vi "Autonomous Independent.vi"() -> ()   [LabVIEW 2016]
doc: "This VI is called when autonomous begins, and will automatically be terminated when autonomous ends. You can carry out timed or sensor driven robot movement independently without needing to return to the caller."
uses:
  <vilib>/Rock Robotics/WPI/Utilities/WPI_GetSetVariantRefNum.vi
  <vilib>/Rock Robotics/Network Tables/NT Read String.vi
  SubSystems/References/Refnums.vi
  <vilib>/Rock Robotics/WPI/RobotDrive/WPI_RobotDriveArcadeDrive_Standard(NoSaturation).vi
  <vilib>/Rock Robotics/Network Tables/NT Write Numeric Array.vi
panel:
  out "Motor Output 2":dbl
  out "Motor Output":dbl
  out "inside timer value 2":u32
  out "Current Movement, for debugging":T1 {"Y Joystick Value" scale=1.0..-1.0; "X Joystick Value" scale=-1.0..1.0}
  in  "Array of robot movements":T2(array[cluster])=[{"X Joystick Value"=0.39393939393939403, "Y Joystick Value"=0.0, "Delay (sec)"=1.0, "Movement Name"="turn"}, {"X Joystick Value"=-0.3737373737373737, "Y Joystick Value"=0.0, "Delay (sec)"=1.0, "Movement Name"="turn back"}] {"Y Joystick Value" scale=1.0..-1.0; "X Joystick Value" scale=-1.0..1.0}
  # "Be sure to right-click and choose Data Operations>>Make Current Value default if you want to save the array values with the VI"
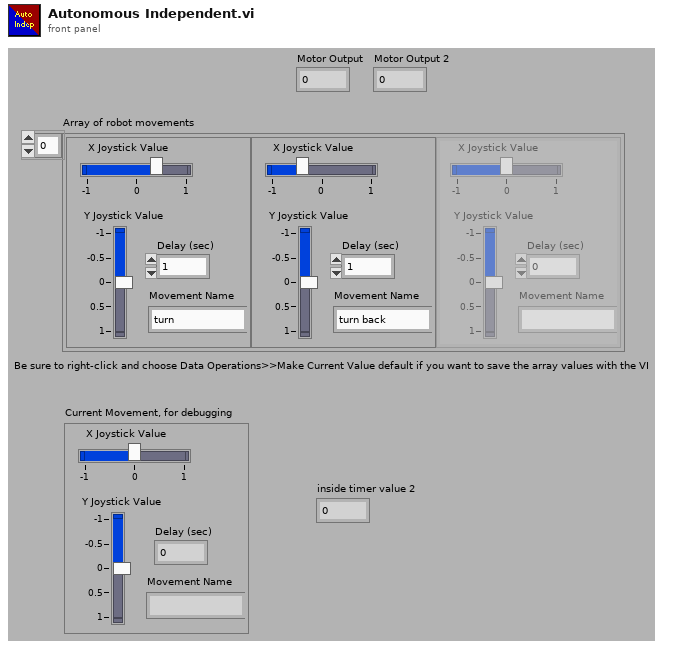
[diagram p1: front panel]
types:
  T1 = cluster{"X Joystick Value":dbl, "Y Joystick Value":dbl, "Delay (sec)":dbl, "Movement Name":string}
  T2 = cluster{"X Joystick Value":dbl, "Y Joystick Value":dbl, "Delay (sec)":dbl, "Movement Name":string}[]
  T3 = typedef "WPI_JoystickDevRef.ctl" = cluster{"Device":T4}
  T4 = typedef "WPI_JoystickDeviceEnum.ctl" = enum16{"USB 0", "USB 1", "USB 2", "USB 3", "USB 4", "USB 5"}
  T5 = typedef "WPI_MotorControlDeviceRef.ctl" = cluster{"DeviceStatus":errorcluster, "Type":T6, "PWM":cluster{"PWM Channel":T7, "DeadBand":T8}, "CAN":cluster{"Device Number":u8, "SetOutput VI Ref":variant, "GetOutput VI Ref":variant, "Enable VI Ref":variant, "Disable VI Ref":variant, "Data":variant}, "Invert":bool}
  T6 = typedef "WPI_MotorControlType.ctl" = enum16{"PWM", "CAN"}
  T7 = typedef "FPGA_DIOPWMChannel.ctl" = enum8{"PWM 0", "PWM 1", "PWM 2", "PWM 3", "PWM 4", "PWM 5", "PWM 6", "PWM 7", "PWM 8", "PWM 9", "PWM MXP 0", "PWM MXP 1", "PWM MXP 2", "PWM MXP 3", "PWM MXP 4", "PWM MXP 5", "PWM MXP 6", "PWM MXP 7", "PWM MXP 8", "PWM MXP 9", "Invalid"}
  T8 = typedef "WPI_PWMDeadband.ctl" = cluster{"Name":string, "maxPositivePwm":i32, "minPositivePwm":i32, "centerPwm":i32, "maxNegativePwm":i32, "minNegativePwm":i32, "angularRange":u16}
  T9 = typedef "WPI_RobotDriveDevRef.ctl" = cluster{"DevStatus":errorcluster, "Motors[]":T5[], "Square Inputs":bool, "Max Output":dbl}
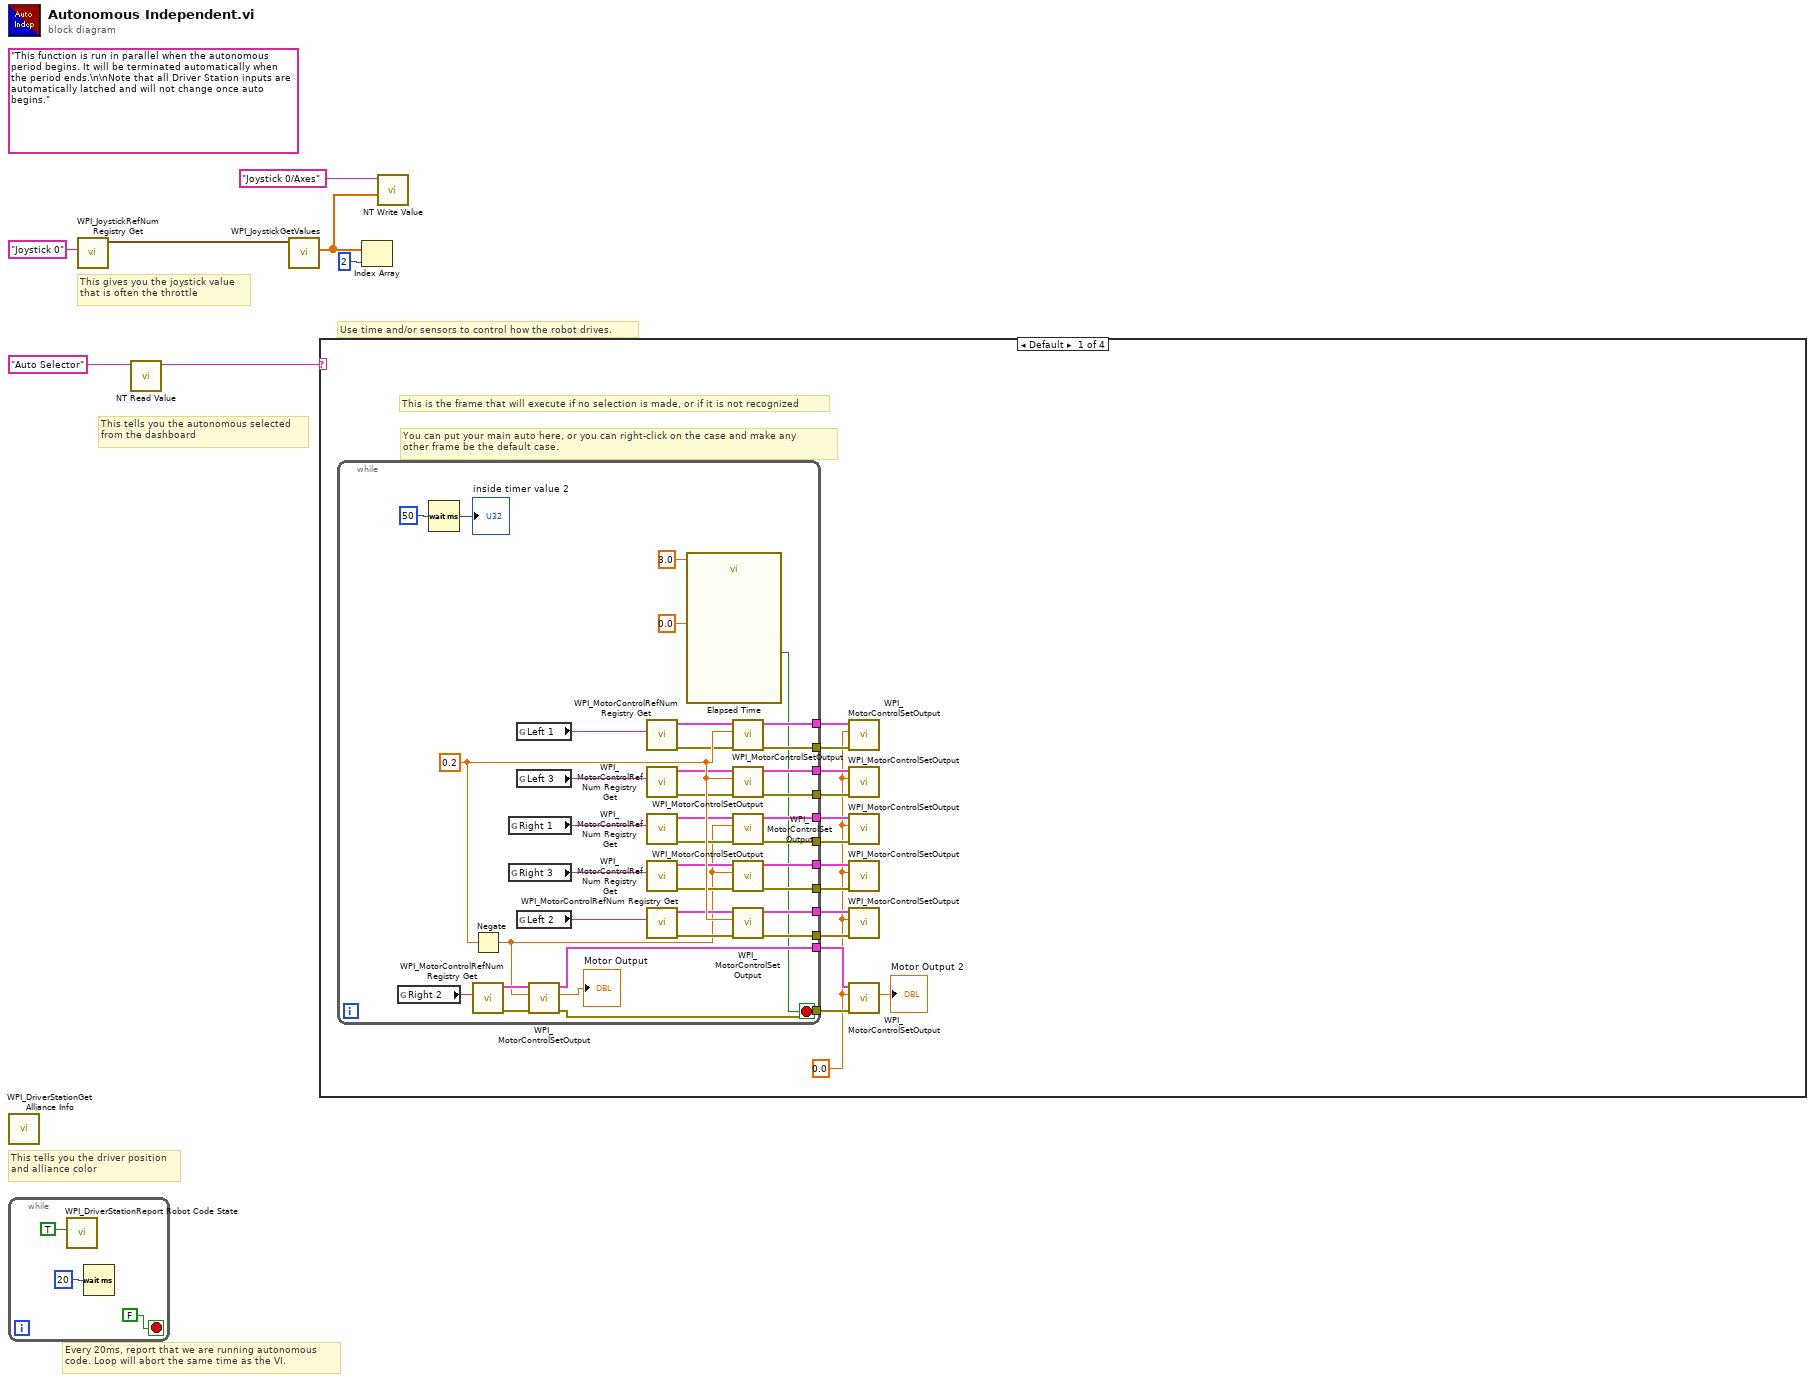
[diagram p0: block diagram]
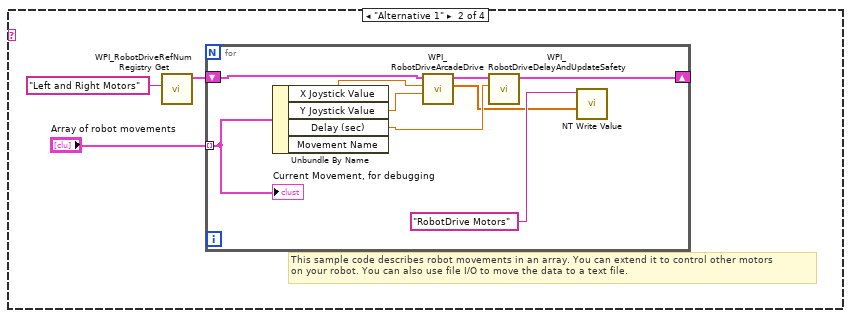
[diagram p2: hidden frame]
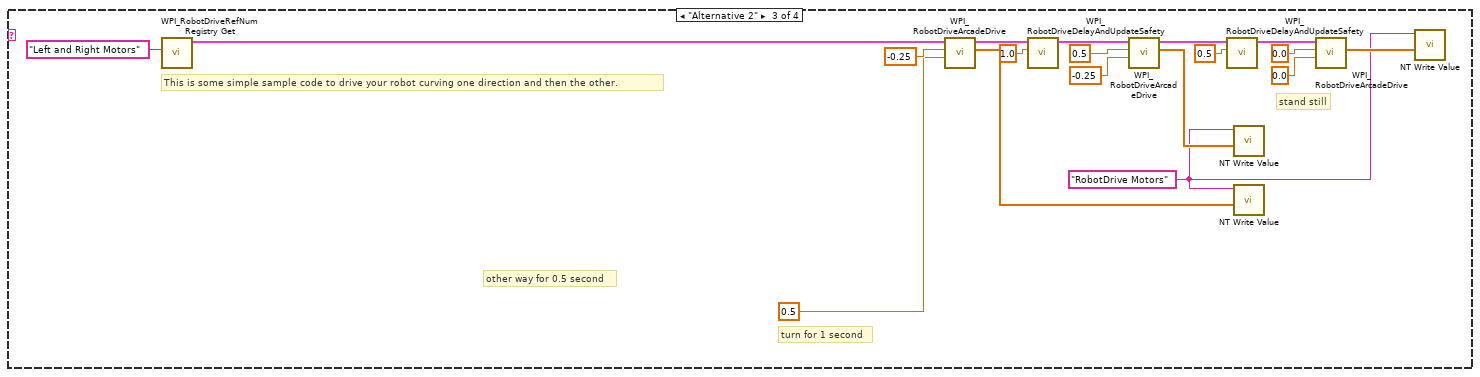
[diagram p3: hidden frame]
diagram:
  (unwired) "This function is run in parallel when the autonomous period begins. It will be terminated automatically when the period ends.\n\nNote that all Driver Station inputs are automatically latched and will not change once auto begins."
  # "This tells you the autonomous selected\nfrom the dashboard"
  # "Every 20ms, report that we are running autonomous\ncode. Loop will abort the same time as the VI."
  # "This gives you the joystick value\nthat is often the throttle"
  # "Use time and/or sensors to control how the robot drives."
  # "This tells you the driver position\nand alliance color"
  n1 = call <vilib>:"WPI_DriverStationGet Alliance Info.vi"() -> ()  [unwired: 12 out]
  n2 = while {
    stop <- FALSE stop-if-true
    n3 = call <vilib>:"WPI_DriverStationReport Robot Code State.vi"("Autonomous"=TRUE) -> ()  [unwired: 10 in, 1 out]
    n4 = Wait (ms)(milliseconds to wait=u32 20) -> ()  [unwired: 1 out]
  }
  n5 = call <vilib>:"WPI_JoystickRefNum Registry Get.vi"("refnum name"="Joystick 0") -> ("JoystickDevRef"=w6:T3)  [unwired: 1 in, 9 out]
  n6 = call-poly <vilib>:"NT Read Value.vi"("Name"="Auto Selector") -> ("String"=w3:string)  [unwired: 9 in, 1 out]
  n7 = call <vilib>:"WPI_JoystickGetValues.vi"("JoystickDevRef"=w6) -> ("Axes"=w2:dbl[])  [unwired: 6 in, 4 out]
  n8 = case shown="Default" w3 {
    frame Default {
      w12 = 0.0 ("Output")
      # "You can put your main auto here, or you can right-click on the case and make any\nother frame be the default case."
      # "This is the frame that will execute if no selection is made, or if it is not recognized"
      n9 = while {
        tunnel: [w40] -> w24
        tunnel: [w39] -> w23
        tunnel: [w38] -> w22
        tunnel: [w37] -> w21
        tunnel: [w36] -> w20
        tunnel: [w35] -> w19
        tunnel: [w34] -> w18
        tunnel: [w33] -> w17
        tunnel: [w32] -> w16
        tunnel: [w31] -> w15
        tunnel: [w30] -> w14
        tunnel: [w29] -> w13
        stop <- w28 stop-if-true
        w61 = 0.2 ("x")
        n10 = global read "Refnums.vi" "Right 2"() -> (w57:string)
        n11 = Wait (ms)(milliseconds to wait=u32 50) -> (millisecond timer value=→"inside timer value 2":u32)
        n12 = Negate(x=w61) -> (-x=w43:dbl)
        n13 = call <vilib>:"WPI_MotorControlRefNum Registry Get.vi"("refnum name"=w57) -> ("error out"=w55:errorcluster, "MotorControlDevRef"=w56:T5)  [unwired: 9 in]
        n14 = global read "Refnums.vi" "Right 1"() -> (w58:string)
        n15 = global read "Refnums.vi" "Right 3"() -> (w52:string)
        n16 = global read "Refnums.vi" "Left 1"() -> (w45:string)
        n17 = global read "Refnums.vi" "Left 3"() -> (w51:string)
        n18 = global read "Refnums.vi" "Left 2"() -> (w46:string)
        n19 = call <vilib>:"WPI_MotorControlSetOutput.vi"("error in (no error)"=w55, "Output"=w43, "MotorControlDevRef"=w56) -> ("error out"=w30:errorcluster, "Motor Output"=→"Motor Output":dbl, "MotorControlDevRef"=w36:T5)  [unwired: 6 in]
        n20 = call <vilib>:"WPI_MotorControlRefNum Registry Get.vi"("refnum name"=w45) -> ("error out"=w44:errorcluster, "MotorControlDevRef"=w42:T5)  [unwired: 9 in]
        n21 = call <vilib>:"WPI_MotorControlRefNum Registry Get.vi"("refnum name"=w51) -> ("error out"=w49:errorcluster, "MotorControlDevRef"=w50:T5)  [unwired: 9 in]
        n22 = call <vilib>:"WPI_MotorControlRefNum Registry Get.vi"("refnum name"=w58) -> ("error out"=w60:errorcluster, "MotorControlDevRef"=w59:T5)  [unwired: 9 in]
        n23 = call <vilib>:"WPI_MotorControlRefNum Registry Get.vi"("refnum name"=w52) -> ("error out"=w54:errorcluster, "MotorControlDevRef"=w53:T5)  [unwired: 9 in]
        n24 = call <vilib>:"WPI_MotorControlRefNum Registry Get.vi"("refnum name"=w46) -> ("error out"=w48:errorcluster, "MotorControlDevRef"=w47:T5)  [unwired: 9 in]
        n25 = call "Elapsed Time"("Time Target (s)"=3.0, "Set Start Time (s)"=0.0) -> ("Time has Elapsed"=w28:bool)  [unwired: 10 in, 7 out]
        n26 = call <vilib>:"WPI_MotorControlSetOutput.vi"("error in (no error)"=w44, "Output"=w61, "MotorControlDevRef"=w42) -> ("error out"=w33:errorcluster, "MotorControlDevRef"=w40:T5)  [unwired: 6 in, 1 out]
        n27 = call <vilib>:"WPI_MotorControlSetOutput.vi"("error in (no error)"=w49, "Output"=w61, "MotorControlDevRef"=w50) -> ("error out"=w34:errorcluster, "MotorControlDevRef"=w38:T5)  [unwired: 6 in, 1 out]
        n28 = call <vilib>:"WPI_MotorControlSetOutput.vi"("error in (no error)"=w60, "Output"=w43, "MotorControlDevRef"=w59) -> ("error out"=w31:errorcluster, "MotorControlDevRef"=w37:T5)  [unwired: 6 in, 1 out]
        n29 = call <vilib>:"WPI_MotorControlSetOutput.vi"("error in (no error)"=w54, "Output"=w43, "MotorControlDevRef"=w53) -> ("error out"=w32:errorcluster, "MotorControlDevRef"=w35:T5)  [unwired: 6 in, 1 out]
        n30 = call <vilib>:"WPI_MotorControlSetOutput.vi"("error in (no error)"=w48, "Output"=w61, "MotorControlDevRef"=w47) -> ("error out"=w29:errorcluster, "MotorControlDevRef"=w39:T5)  [unwired: 6 in, 1 out]
      }
      n31 = call <vilib>:"WPI_MotorControlSetOutput.vi"("error in (no error)"=w17, "Output"=w12, "MotorControlDevRef"=w24) -> ()  [unwired: 6 in, 3 out]
      n32 = call <vilib>:"WPI_MotorControlSetOutput.vi"("error in (no error)"=w18, "Output"=w12, "MotorControlDevRef"=w22) -> ()  [unwired: 6 in, 3 out]
      n33 = call <vilib>:"WPI_MotorControlSetOutput.vi"("error in (no error)"=w15, "Output"=w12, "MotorControlDevRef"=w21) -> ()  [unwired: 6 in, 3 out]
      n34 = call <vilib>:"WPI_MotorControlSetOutput.vi"("error in (no error)"=w16, "Output"=w12, "MotorControlDevRef"=w19) -> ()  [unwired: 6 in, 3 out]
      n35 = call <vilib>:"WPI_MotorControlSetOutput.vi"("error in (no error)"=w13, "Output"=w12, "MotorControlDevRef"=w23) -> ()  [unwired: 6 in, 3 out]
      n36 = call <vilib>:"WPI_MotorControlSetOutput.vi"("error in (no error)"=w14, "Output"=w12, "MotorControlDevRef"=w20) -> ("Motor Output"=→"Motor Output 2":dbl)  [unwired: 6 in, 2 out]
    }
    frame "Alternative 1" {
      # "This sample code describes robot movements in an array. You can extend it to control other motors\non your robot. You can also use file I/O to move the data to a text file."
      n37 = call <vilib>:"WPI_RobotDriveRefNum Registry Get.vi"("refnum name"="Left and Right Motors") -> ("RobotDriveDevRef"=w64:T9)  [unwired: 1 in, 9 out]
      n38 = for {
        shift-right: [w72] -> _
        shift-left: w64 -> [w73]
        tunnel: "Array of robot movements" -> [w68] mode=indexing
        n39 = Unbundle By Name(w68) -> ("X Joystick Value"=w71:dbl, "Y Joystick Value"=w70:dbl, "Delay (sec)"=w69:dbl)  [unwired: 1 out]
        n40 = call-poly <vilib>:"WPI_RobotDriveArcadeDrive.vi"("Y axis value"=w70, "X axis value"=w71, "RobotDriveDevRef"=w73) -> ("Motor Values"=w66:dbl[], "RobotDriveDevRef"=w74:T9)  [unwired: 1 in, 6 out]
        n41 = call <vilib>:"WPI_RobotDriveDelayAndUpdateSafety.vi"("Delay (s)"=w69, "RobotDriveDevRef"=w74) -> ("RobotDriveDevRef 2"=w72:T9)  [unwired: 8 in, 1 out]
        n42 = call-poly <vilib>:"NT Write Value.vi"("Numeric Array"=w66, "Name"="RobotDrive Motors") -> ()  [unwired: 9 in, 1 out]
        "Current Movement, for debugging" <- w68
      }
    }
    frame "Alternative 2" {
      w76 = "RobotDrive Motors" ("Name")
      # "This is some simple sample code to drive your robot curving one direction and then the other."
      # "stand still"
      # "other way for 0.5 second"
      # "turn for 1 second"
      n43 = call <vilib>:"WPI_RobotDriveRefNum Registry Get.vi"("refnum name"="Left and Right Motors") -> ("RobotDriveDevRef"=w92:T9)  [unwired: 1 in, 9 out]
      n44 = call-poly <vilib>:"WPI_RobotDriveArcadeDrive.vi"("Y axis value"=0.5 ("X axis value"), "X axis value"=-0.25, "RobotDriveDevRef"=w92) -> ("Motor Values"=w75:dbl[], "RobotDriveDevRef"=w85:T9)  [unwired: 1 in, 6 out]
      n45 = call <vilib>:"WPI_RobotDriveDelayAndUpdateSafety.vi"("Delay (s)"=1.0, "RobotDriveDevRef"=w85) -> ("RobotDriveDevRef 2"=w86:T9)  [unwired: 8 in, 1 out]
      n46 = call-poly <vilib>:"WPI_RobotDriveArcadeDrive.vi"("Y axis value"=-0.25 ("X axis value"), "X axis value"=0.5, "RobotDriveDevRef"=w86) -> ("Motor Values"=w77:dbl[], "RobotDriveDevRef"=w87:T9)  [unwired: 1 in, 6 out]
      n47 = call <vilib>:"WPI_RobotDriveDelayAndUpdateSafety.vi"("Delay (s)"=0.5, "RobotDriveDevRef"=w87) -> ("RobotDriveDevRef 2"=w88:T9)  [unwired: 8 in, 1 out]
      n48 = call-poly <vilib>:"NT Write Value.vi"("Numeric Array"=w77, "Name"=w76) -> ()  [unwired: 9 in, 1 out]
      n49 = call-poly <vilib>:"NT Write Value.vi"("Numeric Array"=w75, "Name"=w76) -> ()  [unwired: 9 in, 1 out]
      n50 = call-poly <vilib>:"WPI_RobotDriveArcadeDrive.vi"("Y axis value"=0.0 ("X axis value"), "X axis value"=0.0, "RobotDriveDevRef"=w88) -> ("Motor Values"=w78:dbl[])  [unwired: 1 in, 7 out]
      n51 = call-poly <vilib>:"NT Write Value.vi"("Numeric Array"=w78, "Name"=w76) -> ()  [unwired: 9 in, 1 out]
    }
    frame "Your Turn" {
    }
  }
  n52 = Index Array(array=w2, index=2) -> ()  [unwired: 1 out]
  n53 = call-poly <vilib>:"NT Write Value.vi"("Numeric Array"=w2, "Name"="Joystick 0/Axes") -> ()  [unwired: 9 in, 1 out]
